vi "Convert Response Type.vi"(8 "error in (no error)":errorcluster, 10 "Response Type String (\"\")":string, 11 "VISA resource name":refnum<visa-resource-name>) -> (0 "error out":errorcluster, 1 "Response Type":i32(ring) items=["Affirmative", "Single Negative", "Multiple Negative", "ASCII", "Binary", "End"], 3 "VISA resource name out":refnum<visa-resource-name>)   [LabVIEW 2011, in "Yokogawa DX Series.lvlib"]
doc: "This VI converts 1 character to a value as response type."
uses:
  <instrlib>/Yokogawa DX Series/Yokogawa DX Series.lvlib
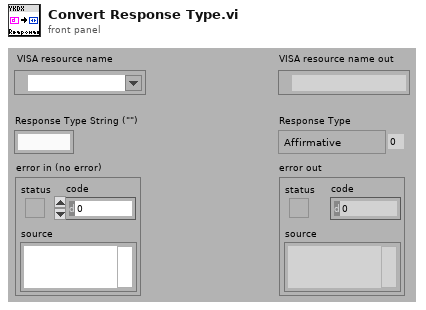
[diagram p1: front panel]
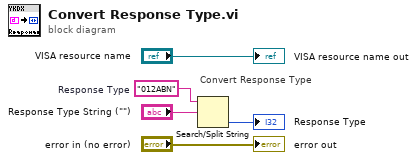
[diagram p0: block diagram]
diagram:
  w2 = "012ABN"  # Response Type
  # "Convert Response Type"
  n1 = Search/Split String(string=w2, search string/char (-)="Response Type String (\"\")") -> (offset of match=→"Response Type":i32)  [unwired: 3 out]
  "VISA resource name out" <- "VISA resource name"
  "error out" <- "error in (no error)"
